vi "FilterByProductID.vi"() -> ()   [LabVIEW 2009]
uses:
  C:/Samples/LabVIEW/FilterByProductID/LabVIEW 2009/UsbDllWrap.dll
panel:
  out "Output:":string
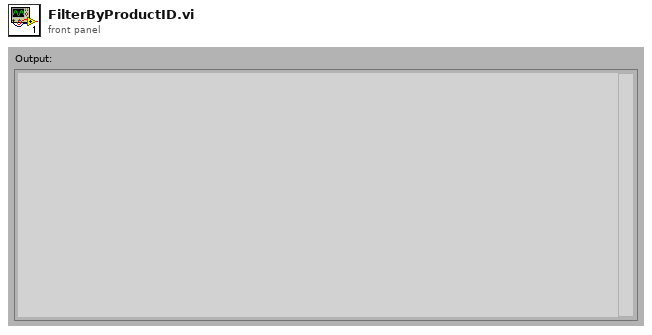
[diagram p1: front panel]
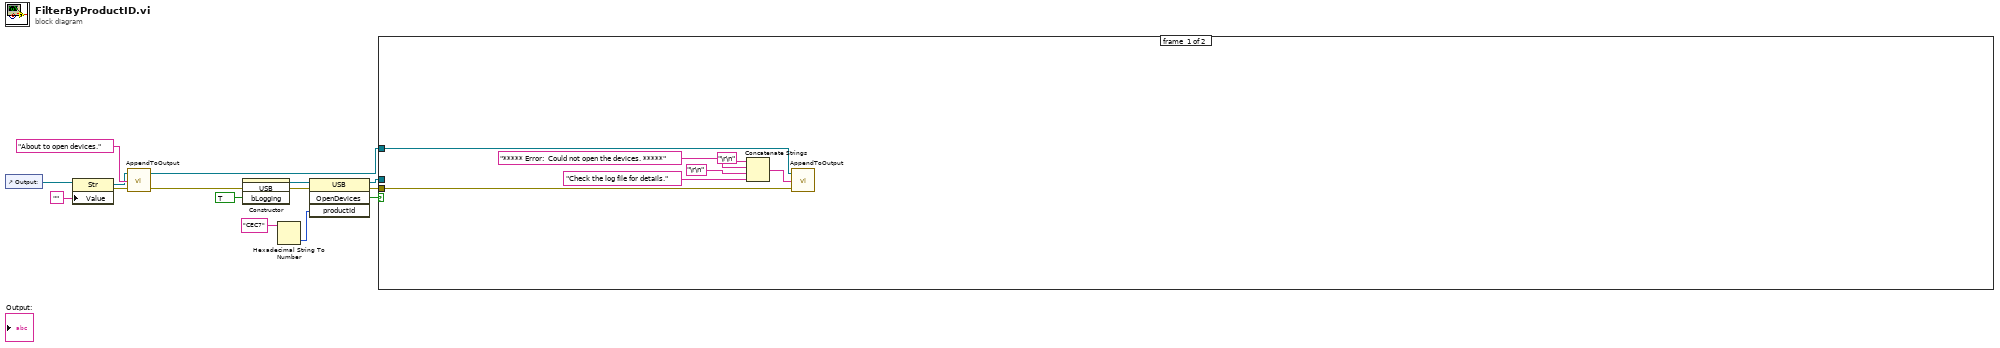
[diagram p0: block diagram]
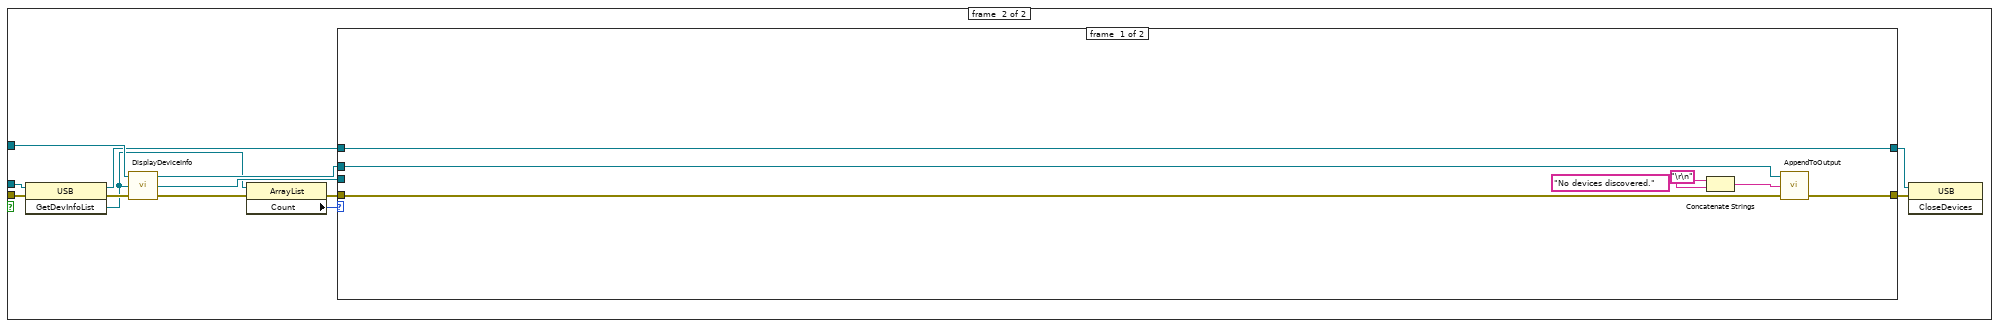
[diagram p2: hidden frame]
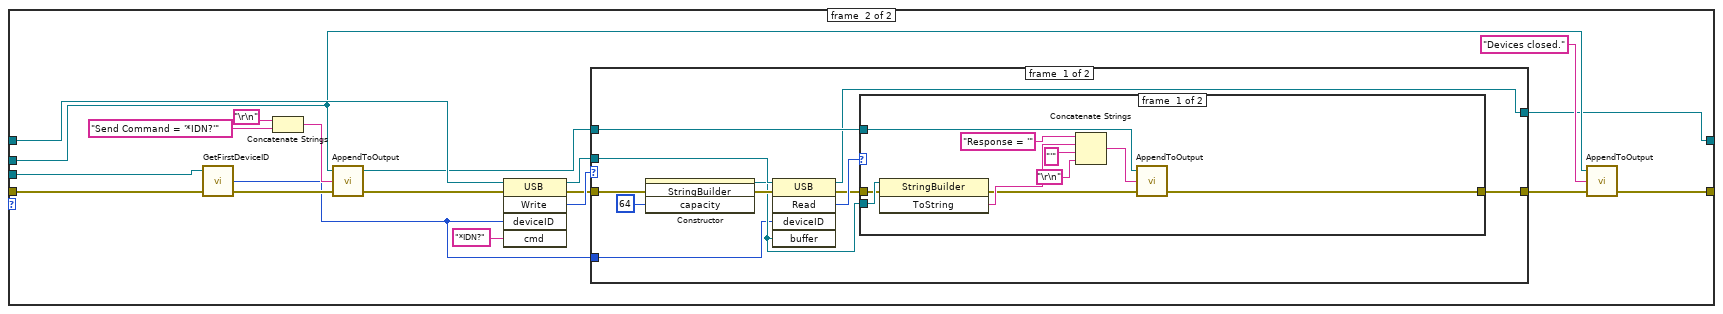
[diagram p3: hidden frame]
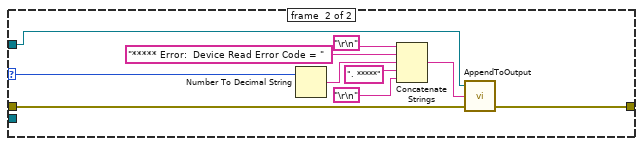
[diagram p4: hidden frame]
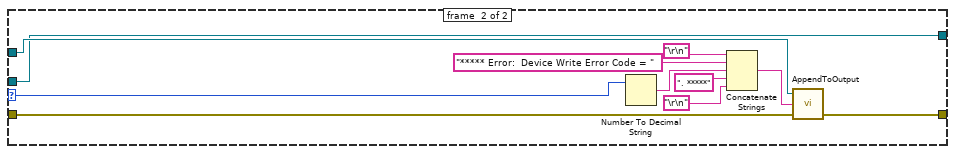
[diagram p5: hidden frame]
diagram:
  n1 = control-ref of="Output:"() -> (w6:refnum<vi>)
  n2 = property class="Str"(reference=w6, "Value"="") -> (reference out=w3:refnum<vi>, error out=w4:errorcluster)  [unwired: 1 in]
  n3 = call "AppendToOutput.vi"("error in"=w4, "Input String"="About to open devices.", "Output Refnum In"=w3) -> ("error out"=w13:errorcluster, "Output Refnum Out"=w10:refnum<vi>)  [unwired: 1 in]
  n4 = constructor class="USB"(error in=w13, "bLogging"=TRUE) -> (reference out=w12:refnum<k24>, error out=w9:errorcluster)  [unwired: 2 in, 2 out]
  n5 = Hexadecimal String To Number(string="CEC7") -> (number=w1:u32)  [unwired: 2 in, 1 out]
  n6 = invoke class="USB" method="OpenDevices"(reference=w12, error in=w9, "productId"=w1) -> (reference out=w7:refnum<k24>, error out=w8:errorcluster, "OpenDevices"=w11:bool)  [unwired: 1 in, 1 out]
  n7 = case shown="True" w11 {
    tunnel: w10 -> [w22 w33]
    tunnel: w8 -> [w21 w34]
    tunnel: w7 -> [_ w35]
    frame #0 {
      n8 = Concatenate Strings("\r\n", "***** Error:  Could not open the devices. *****", "\r\n", "Check the log file for details.") -> (w17:string)
      n9 = call "AppendToOutput.vi"("error in"=w21, "Input String"=w17, "Output Refnum In"=w22) -> ()  [unwired: 1 in, 2 out]
    }
    frame #1 {
      n10 = invoke class="USB" method="GetDevInfoList"(reference=w35, error in=w34) -> (reference out=w31:refnum<k24>, error out=w32:errorcluster, "GetDevInfoList"=w26:refnum<k24>)  [unwired: 1 in]
      n11 = call "DisplayDeviceInfo.vi"("error in"=w32, "DevInfoList In"=w26, "Output Refnum In"=w33) -> ("error out"=w23:errorcluster, "DevInfoList Out"=w30:refnum<k24>, "Output Refnum Out"=w29:refnum<vi>)
      n12 = property class="ArrayList"(reference=w26, error in=w23) -> (error out=w24:errorcluster, "Count"=w25:i32)  [unwired: 1 out]
      n13 = case shown="1, Default" w25 {
        tunnel: w31 -> [w36 w57]
        tunnel: w24 -> [w39 w55]
        tunnel: w30 -> [_ w54]
        tunnel: w29 -> [w38 w47]
        tunnel: [w37 w44] -> w28
        tunnel: [w36 w43] -> w27
        frame #0 {
          n14 = Concatenate Strings("\r\n", "No devices discovered." ("string")) -> (w40:string)
          n15 = call "AppendToOutput.vi"("error in"=w39, "Input String"=w40, "Output Refnum In"=w38) -> ("error out"=w37:errorcluster)  [unwired: 1 in, 1 out]
        }
        frame #1 {
          n16 = call "GetFirstDeviceID.vi"("error in"=w55, "DevInfoList In"=w54) -> ("error out"=w53:errorcluster, "Device ID"=w45:i32)  [unwired: 1 in, 1 out]
          n17 = Concatenate Strings("\r\n", "Send Command = '*IDN?'") -> (w59:string)
          n18 = call "AppendToOutput.vi"("error in"=w53, "Input String"=w59, "Output Refnum In"=w47) -> ("error out"=w56:errorcluster, "Output Refnum Out"=w49:refnum<vi>)  [unwired: 1 in]
          n19 = invoke class="USB" method="Write"(reference=w57, error in=w56, "deviceID"=w45, "cmd"="*IDN?") -> (reference out=w51:refnum<k24>, error out=w50:errorcluster, "Write"=w52:i32)  [unwired: 1 in, 2 out]
          n20 = case shown="0" w52 {
            selector: w52 -> [_ w98]
            tunnel: w51 -> [w72 w93]
            tunnel: w50 -> [w69 w96]
            tunnel: [w65 w95] -> w46
            tunnel: w49 -> [w64 w94]
            tunnel: w45 -> [w63 _]
            tunnel: [w62 w93] -> w43
            frame #0 {
              n21 = constructor class="StringBuilder"(error in=w69, "capacity"=64) -> (reference out=w67:refnum<k24>, error out=w70:errorcluster)  [unwired: 2 in, 2 out]
              n22 = invoke class="USB" method="Read"(reference=w72, error in=w70, "deviceID"=w63, "buffer"=w67) -> (reference out=w62:refnum<k24>, error out=w66:errorcluster, "Read"=w68:i32)  [unwired: 1 in, 2 out]
              n23 = case shown="0" w68 {
                selector: w68 -> [_ w87]
                tunnel: w67 -> [w82 _]
                tunnel: w66 -> [w81 w84]
                tunnel: [w74 w83] -> w65
                tunnel: w64 -> [w73 w85]
                frame #0 {
                  n24 = invoke class="StringBuilder" method="ToString"(reference=w82, error in=w81) -> (error out=w75:errorcluster, "ToString"=w78:string)  [unwired: 1 in, 1 out]
                  n25 = Concatenate Strings("Response = '", w78, "'", "\r\n") -> (w76:string)
                  n26 = call "AppendToOutput.vi"("error in"=w75, "Input String"=w76, "Output Refnum In"=w73) -> ("error out"=w74:errorcluster)  [unwired: 1 in, 1 out]
                }
                frame #1 {
                  n27 = Number To Decimal String(number=w87) -> (decimal integer string=w92:string)  [unwired: 1 in]
                  n28 = Concatenate Strings("\r\n", "***** Error:  Device Read Error Code = ", w92, ". *****", "\r\n") -> (w86:string)
                  n29 = call "AppendToOutput.vi"("error in"=w84, "Input String"=w86, "Output Refnum In"=w85) -> ("error out"=w83:errorcluster)  [unwired: 1 in, 1 out]
                }
              }
            }
            frame #1 {
              n30 = Number To Decimal String(number=w98) -> (decimal integer string=w99:string)  [unwired: 1 in]
              n31 = Concatenate Strings("\r\n", "***** Error:  Device Write Error Code = ", w99, ". *****", "\r\n") -> (w97:string)
              n32 = call "AppendToOutput.vi"("error in"=w96, "Input String"=w97, "Output Refnum In"=w94) -> ("error out"=w95:errorcluster)  [unwired: 1 in, 1 out]
            }
          }
          n33 = call "AppendToOutput.vi"("error in"=w46, "Input String"="Devices closed." ("string"), "Output Refnum In"=w47) -> ("error out"=w44:errorcluster)  [unwired: 1 in, 1 out]
        }
      }
      n34 = invoke class="USB" method="CloseDevices"(reference=w27, error in=w28) -> ()  [unwired: 1 in, 3 out]
    }
  }
